vi "Add Line.vi"(8 "error in (no error)":errorcluster, 10 "Line":T1, 11 "user control module configuration in":refnum<class "user control module configuration.lvclass">) -> (0 "error out":errorcluster, 3 "user control module configuration out":refnum<class "user control module configuration.lvclass">)   [LabVIEW 2013, in "user control module configuration.lvclass"]
uses:
  user control module configuration.lvclass
  <vilib>/NI/Tag Bus Module Framework/channel/TBM channel.lvclass
  user control module configuration.lvclass/user control module configuration.ctl
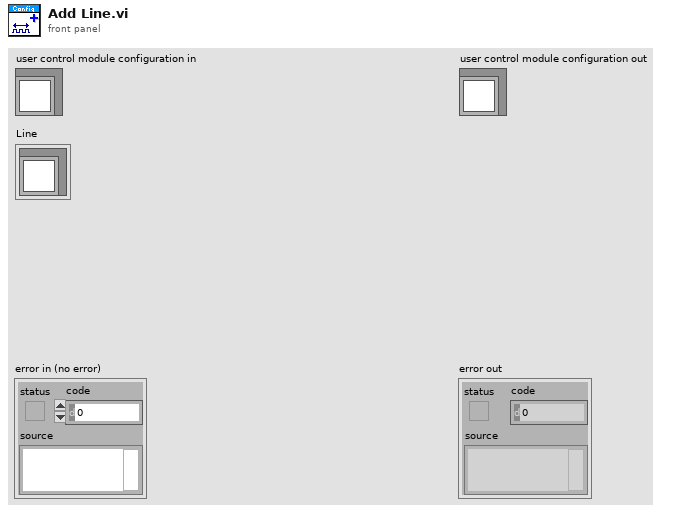
[diagram p1: front panel]
types:
  T1 = cluster{"channel":refnum<class "TBM channel.lvclass">}
  T2 = cluster{"channel":refnum<class "TBM channel.lvclass">}[]
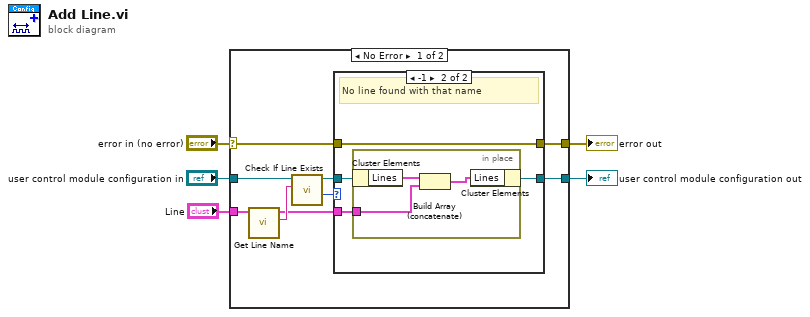
[diagram p0: block diagram]
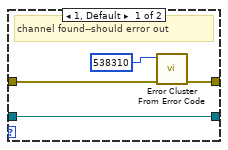
[diagram p2: hidden frame]
diagram:
  n1 = case shown="No Error" "error in (no error)" {
    selector: "error in (no error)" -> [w8 w27]
    tunnel: [w7 w27] -> w4
    tunnel: [w6 w26] -> w2
    tunnel: "user control module configuration in" -> [w12 w26]
    tunnel: "Line" -> [w14 _]
    frame No Error {
      n2 = call "Get Line Name.vi"("Line in"=w14) -> ("Name"=w13:string, "Line out"=w10:T1)  [unwired: 8 in, 1 out]
      n3 = call-dynamic "Check If Line Exists.vi"("name to locate"=w13, "user control module configuration in"=w12) -> ("index"=w9:i32, "user control module configuration out"=w11:refnum<class "user control module configuration.lvclass">)  [unwired: 5 in, 3 out]
      n4 = case shown="-1" w9 {
        tunnel: [w18 w21] -> w7
        tunnel: w8 -> [w16 w21]
        tunnel: w11 -> [w15 w20]
        tunnel: w10 -> [_ w22]
        tunnel: [w15 w19] -> w6
        frame 1, Default {
          # "channel found--should error out"
          n5 = call <vilib>:"Error Cluster From Error Code.vi"("error in (no error)"=w16, "error code (0)"=538310) -> ("error out"=w18:errorcluster)  [unwired: 7 in]
        }
        frame -1 {
          # "No line found with that name"
          n6 = in-place {
            in-place-border: w22 -> [w23]
            n7 = in-place-cluster #1(w20) -> ("Lines"=w24:T2)
            n8 = Build Array (concatenate)(w24, w23) -> (w25:T2)
            n9 = in-place-cluster #1("Lines"=w25) -> (w19:refnum<class "user control module configuration.lvclass">)
          }
        }
      }
    }
    frame Error {
    }
  }
  "error out" <- w4
  "user control module configuration out" <- w2
